vi "findCorrectionPolynom.vi"(6 "freq":dbl=1.0 format="%#_13g", 8 "error in (no error)":errorcluster, 9 "Range":dbl, 10 "Offset":dbl, 11 "BestThetaLambdaMeanln10f":T1={"Theta"=[-1.0, 1.0, 0.0, 0.0, 0.0, 0.0, 0.0, 0.0, 0.0], "Lambda"=[0.0, 0.0, 0.0, 0.0, 0.0, 0.0, 0.0, 0.0, 0.0], "meanln10f"=0.0}) -> (0 "error out":errorcluster, 1 "Range in micron":dbl, 2 "Polynomial Coefficients Trace":dbl[](array[numeric]))   [LabVIEW 2016]
uses:
  <vilib>/Analysis/NI_AALPro.lvlib
panel:
  out "Voltage=g(pos)":cluster{dbl[], dbl[]}(graph)
  out "pos=f(volt)":cluster{dbl[], dbl[]}(graph)
  in  "Nb PointV2":i32=51
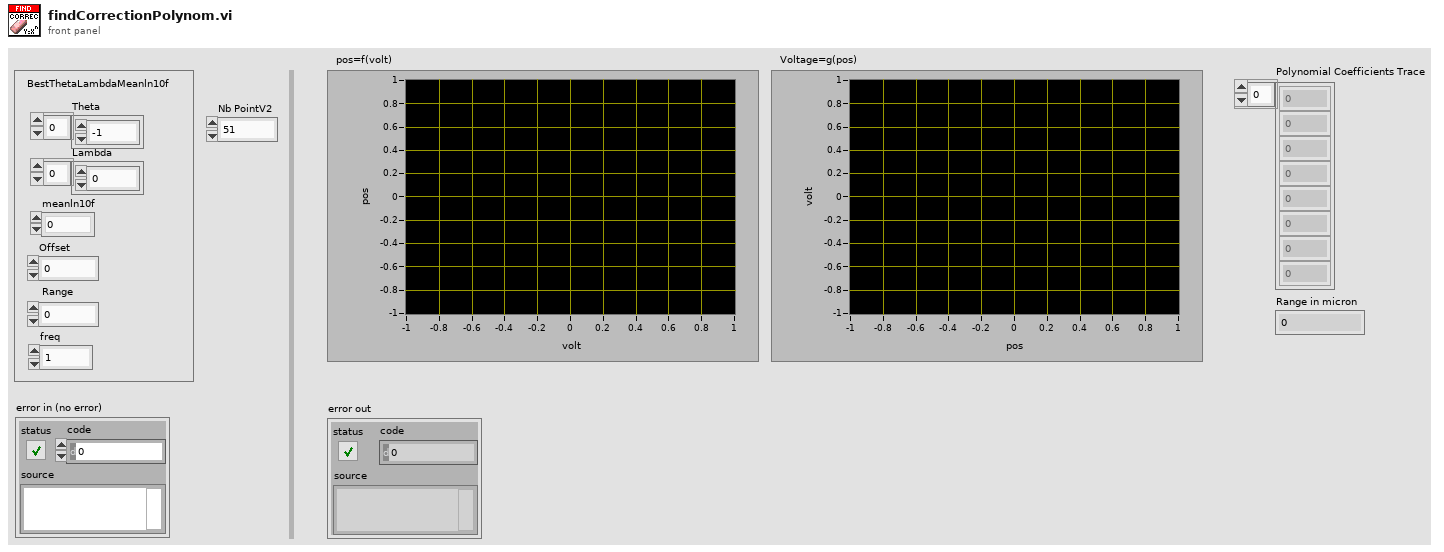
[diagram p1: front panel]
types:
  T1 = cluster{"Theta":dbl[], "Lambda":dbl[], "meanln10f":dbl}
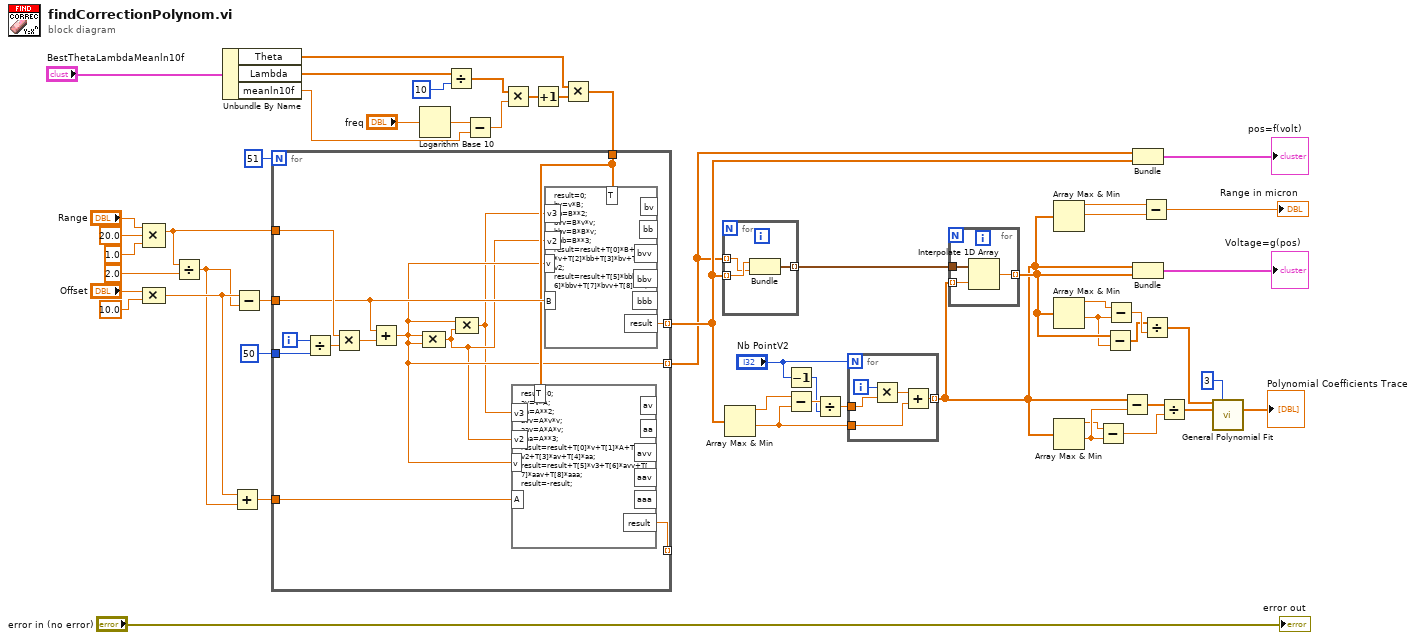
[diagram p0: block diagram]
diagram:
  n1 = Compound Arithmetic op=MULTIPLY("Range", 20.0 ("value"), 1.0 ("value")) -> (w21:dbl)
  n2 = Compound Arithmetic op=MULTIPLY("Offset", 10.0 ("value")) -> (w9:dbl)
  n3 = Divide(x=w21, y=2.0) -> (x/y=w8:dbl)
  n4 = Unbundle By Name("BestThetaLambdaMeanln10f") -> ("Theta"=w4:dbl[], "Lambda"=w3:dbl[], "meanln10f"=w2:dbl)
  n5 = Add(x=w9, y=w8) -> (x+y=w7:dbl)
  n6 = Subtract(x=w9, y=w8) -> (x-y=w28:dbl)
  n7 = Logarithm Base 10(1:"freq") -> (0:w14:dbl)
  n8 = Divide(x=w3, y=10 ("Numeric")) -> (x/y=w11:dbl[])
  n9 = Subtract(x=w14, y=w2) -> (x-y=w15:dbl)
  n10 = Multiply(x=w11, y=w15) -> (x*y=w16:dbl[])
  n11 = Increment(x=w16) -> (x+1=w17:dbl[])
  n12 = Multiply(x=w4, y=w17) -> (x*y=w12:dbl[])
  n13 = for {
    N: 51 -> [_]
    tunnel: w12 -> [w61]
    tunnel: w28 -> [w63]
    tunnel: w21 -> [w65]
    tunnel: [w60] -> w24 mode=indexing
    tunnel: [w62] -> w25 mode=indexing
    tunnel: w7 -> [w57]
    tunnel: [w56] -> _ mode=indexing
    tunnel: 50 ("y") -> [w55]
    i -> [w67]
    n14 = Divide(x=w67, y=w55) -> (x/y=w66:dbl)
    n15 = Multiply(x=w65, y=w66) -> (x*y=w64:dbl)
    n16 = Add(x=w63, y=w64) -> (x+y=w60:dbl)
    n17 = Compound Arithmetic op=MULTIPLY(w60, w60) -> (w59:dbl)
    n18 = Compound Arithmetic op=MULTIPLY(w60, w59) -> (w58:dbl)
    n19 = formula code="result=0;\nav=v*A;\naa=A**2;\navv=A*v*v;\naav=A*A*v;\naaa=A**3;\nresult=result+T[0]*v+T[1]*A+T[2]*v2+T[3]*av+T[4]*aa;\nresult=result+T[5]*v3+T[6]*avv+T[7]*aav+T[8]*aaa;\nresult=-result;"("v"=w60, "A"=w57, "T"=w61, "v2"=w59, "v3"=w58) -> ("result"=w56:dbl)  [unwired: 5 out]
    n20 = formula code="result=0;\nbv=v*B;\nbb=B**2;\nbvv=B*v*v;\nbbv=B*B*v;\nbbb=B**3;\nresult=result+T[0]*B+T[1]*v+T[2]*bb+T[3]*bv+T[4]*v2;\nresult=result+T[5]*bbb+T[6]*bbv+T[7]*bvv+T[8]*v3;"("v"=w60, "B"=w63, "T"=w61, "v2"=w59, "v3"=w58) -> ("result"=w62:dbl)  [unwired: 5 out]
  }
  n21 = for {
    tunnel: w24 -> [w68] mode=indexing
    tunnel: w25 -> [w69] mode=indexing
    tunnel: [w70] -> w54 mode=indexing
    n22 = Bundle("result"=w69, w68) -> (w70:cluster{"result":dbl, dbl})  [unwired: 1 in]
  }
  n23 = Array Max & Min(array=w25) -> (max value=w52:dbl, min value=w53:dbl)  [unwired: 2 out]
  n24 = Decrement(x="Nb PointV2") -> (x-1=w49:i32)
  n25 = Subtract(x=w52, y=w53) -> (x-y=w50:dbl)
  n26 = Divide(x=w50, y=w49) -> (x/y=w51:dbl)
  n27 = for {
    N: "Nb PointV2" -> [_]
    tunnel: w53 -> [w74]
    tunnel: w51 -> [w73]
    tunnel: [w71] -> w34 mode=indexing
    i -> [w72]
    n28 = Multiply(x=w72, y=w73) -> (x*y=w75:dbl)
    n29 = Add(x=w75, y=w74) -> (x+y=w71:dbl)
  }
  n30 = for {
    tunnel: w54 -> [w78]
    tunnel: w34 -> [w77] mode=indexing
    tunnel: [w76] -> w44 mode=indexing
    n31 = Interpolate 1D Array(1:w77, 2:w78) -> (0:w76:dbl)
  }
  n32 = Array Max & Min(array=w34) -> (max value=w32:dbl, min value=w33:dbl)  [unwired: 2 out]
  n33 = Array Max & Min(array=w44) -> (max value=w45:dbl, min value=w43:dbl)  [unwired: 2 out]
  n34 = Array Max & Min(array=w34) -> (max value=w36:dbl, min value=w37:dbl)  [unwired: 2 out]
  n35 = Subtract(x=w36, y=w37) -> (x-y=w38:dbl)
  n36 = Subtract(x=w44, y=w43) -> (x-y=w41:dbl[])
  n37 = Subtract(x=w45, y=w43) -> (x-y=w42:dbl)
  n38 = Subtract(x=w34, y=w37) -> (x-y=w39:dbl[])
  n39 = Bundle(w24, w25) -> (→"pos=f(volt)":cluster{dbl[], dbl[]})  [unwired: 1 in]
  n40 = Bundle(w34, w44) -> (→"Voltage=g(pos)":cluster{dbl[], dbl[]})  [unwired: 1 in]
  n41 = Subtract(x=w32, y=w33) -> (x-y=→"Range in micron":dbl)
  n42 = Divide(x=w41, y=w42) -> (x/y=w40:dbl[])
  n43 = Divide(x=w39, y=w38) -> (x/y=w35:dbl[])
  n44 = call <vilib>:"General Polynomial Fit.vi"("Y"=w40, "polynomial order"=3, "X"=w35) -> ("Polynomial Coefficients"=→"Polynomial Coefficients Trace":dbl[])  [unwired: 9 in, 3 out]
  "error out" <- "error in (no error)"
